vi "Read Variable (String).vi"(8 "error in":errorcluster, 10 "Variable Name":string, 11 "Spark Reference In":T1) -> (0 "error out":errorcluster, 2 "value":string, 3 "Spark Reference Out":T1)   [LabVIEW 2014, in "Spark API.lvlib"]
doc: "Reads Spark registered variables and converts them to the relevant type (string)."
uses:
  Spark API.lvlib
  Controls/Spark Reference.ctl
  <vilib>/httpClient/ClientHandle.ctl
  Controls/Device Query JSON.ctl
  <vilib>/httpClient/LabVIEWHTTPClient.lvlib
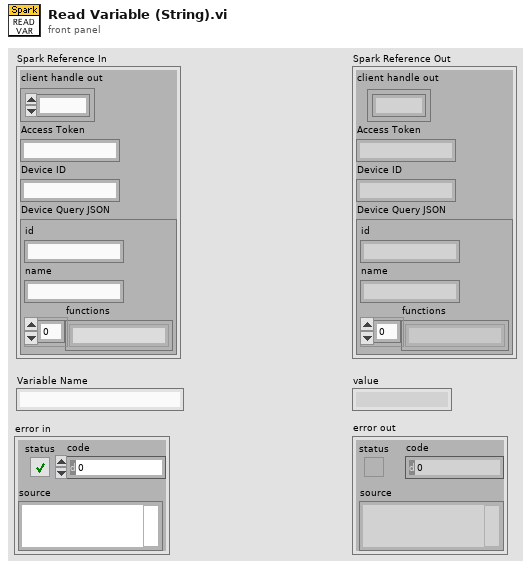
[diagram p1: front panel]
types:
  T1 = typedef "Spark API.lvlib/Spark Reference.ctl" = cluster{"client handle out":T2, "Access Token":string, "Device ID":string, "Device Query JSON":T3}
  T2 = typedef "LabVIEWHTTPClient.lvlib/ClientHandle.ctl" = refnum<k1>
  T3 = typedef "Spark API.lvlib/Device Query JSON.ctl" = cluster{"id":string, "name":string, "functions":string[]}
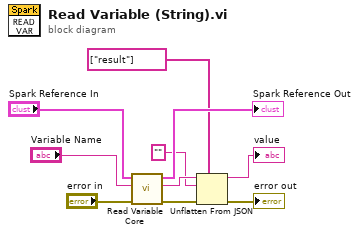
[diagram p0: block diagram]
diagram:
  n1 = call "Read Variable Core.vi"("error in"="error in", "Variable Name"="Variable Name", "Spark Reference In"="Spark Reference In") -> ("error out"=w5:errorcluster, "Variable Response"=w3:string, "Spark Reference Out"=→"Spark Reference Out":T1)  [unwired: 6 in]
  n2 = Unflatten From JSON(path=string[] ["result"], JSON string=w3, type and defaults="", error in (no error)=w5) -> (value=→"value":string, error out=→"error out":errorcluster)  [unwired: 3 in]
